vi "5302GetPhase.vi"(8 "error in (no error)":errorcluster, 11 "VISA Resource Name":refnum<visa-resource-name>) -> (0 "error out":errorcluster, 1 "data string":string, 2 "Phase":dbl format="%.4f", 3 "VISA Resource Name Out":refnum<visa-resource-name>)   [LabVIEW 2015]
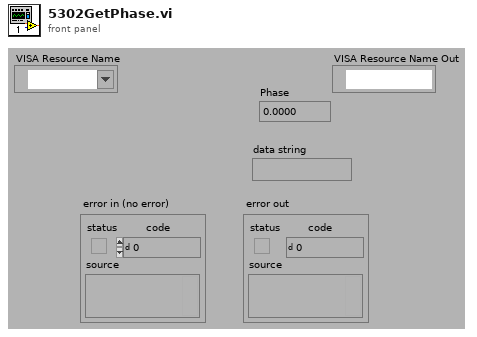
[diagram p1: front panel]
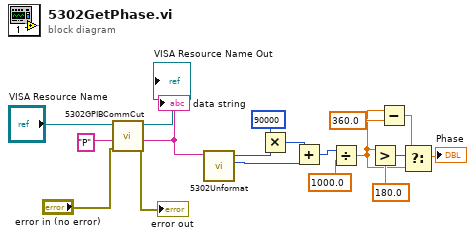
[diagram p0: block diagram]
diagram:
  n1 = call "5302GPIBCommCut.vi"("error in (no error)"="error in (no error)", "data string in"="P" ("data string"), "VISA Resource Name"="VISA Resource Name") -> ("error out"=→"error out":errorcluster, "data string out"=w3:string, "VISA Resource Name Out"=→"VISA Resource Name Out":refnum<visa-resource-name>)  [unwired: 2 in, 4 out]
  "data string" <- w3
  n2 = call "5302Unformat.vi"("Data String"=w3) -> ("Numeric 2"=w4:i32, "Numeric 1"=w5:i32)  [unwired: 9 out]
  n3 = Multiply(x=90000 ("y"), y=w5) -> (x*y=w13:i32)
  n4 = Add(x=w13, y=w4) -> (x+y=w15:i32)
  n5 = Divide(x=w15, y=1000.0) -> (x/y=w7:dbl)
  n6 = Greater?(x=w7, y=180.0) -> (0:w10:bool)
  n7 = Subtract(x=w7, y=360.0) -> (x-y=w8:dbl)
  n8 = Select(t=w8, s=w10, f=w7) -> (s? t:f=→"Phase":dbl)
